vi "Data Listener.vi"(8 "error in":errorcluster, 10 "Data":T1, 11 "Connection ID":u64) -> (0 "error out":errorcluster)   [LabVIEW 2015, in "Front Panel Publisher.lvlib" / "Websocket.lvclass"]
uses:
  Websocket.lvclass
  Private/Connection Data.ctl
  Private/Mask.vi
  <vilib>/wsapi/VIs/Unescape HTTP URL.vi
  Front Panel Manager_class/FP Server Set Data.vi
  Front Panel Manager_class/FP Server Get Data.vi
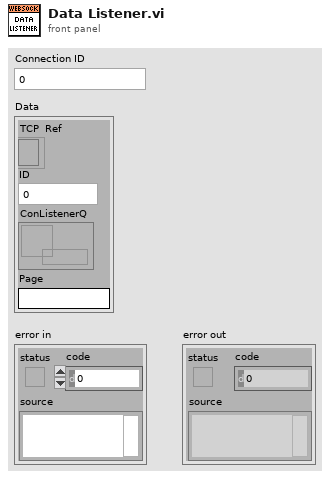
[diagram p1: front panel]
types:
  T1 = typedef "Front Panel Publisher.lvlib/Websocket.lvclass/Connection Data.ctl" = cluster{"TCP  Ref":refnum<k5>, "connection ID":u64, "ConListenerQ":refnum<queue>, "Page":string}
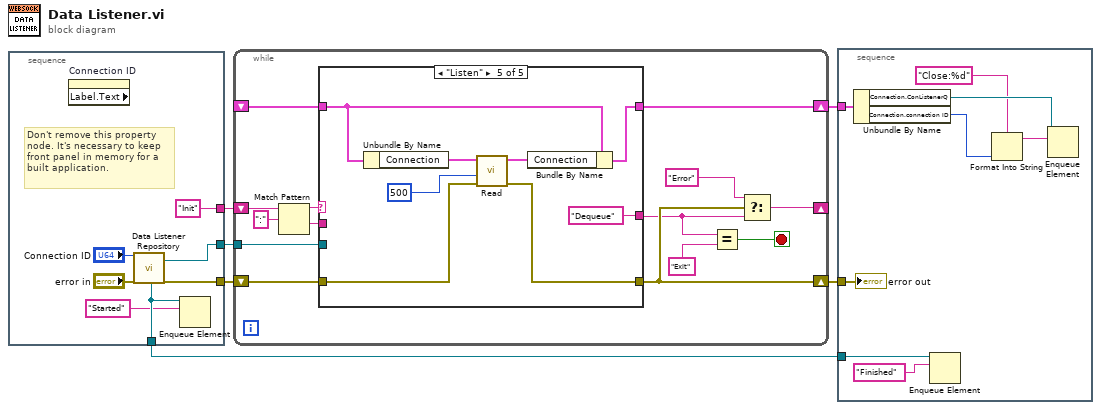
[diagram p0: block diagram]
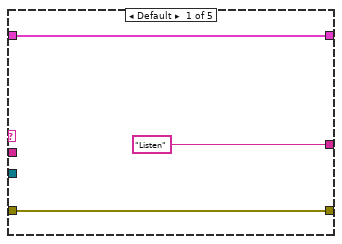
[diagram p2: hidden frame]
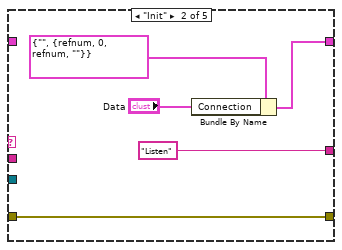
[diagram p3: hidden frame]
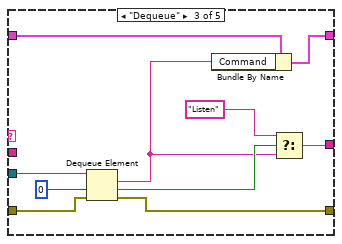
[diagram p4: hidden frame]
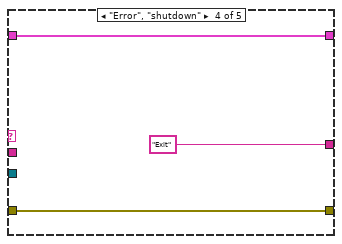
[diagram p5: hidden frame]
diagram:
  n1 = stacked-sequence {
    tunnel: [w11] -> w6
    tunnel: [w10] -> w4
    tunnel: [w8] -> w3
    tunnel: ["Init"] -> w2
    frame #0 {
      # "Don't remove this property node. It's necessary to keep front panel in memory for a built application."
      n2 = property on="Connection ID" class="DigNum (strict)" props=["Label", "Text"]() -> ()  [unwired: 2 in, 3 out]
      n3 = call "Data Listener Repository.vi"("Connection ID"="Connection ID", "error in (no error)"="error in") -> ("ProcessSyncQueue"=w8:refnum<queue>, "ToProcessQueue"=w10:refnum<queue>, "error out"=w11:errorcluster)  [unwired: 12 in, 3 out]
      n4 = Enqueue Element(queue=w8, element="Started") -> ()  [unwired: 2 in, 3 out]
    }
  }
  n5 = while {
    shift-right: [w22] -> w5
    shift-left: w6 -> [w14]
    tunnel: w4 -> [w27]
    shift-right: [w20] -> _
    shift-left: w2 -> [w25]
    shift-right: [w16] -> w1
    shift-left: _ -> [w15]
    stop <- w17 stop-if-true
    n6 = Match Pattern(string=w25, regular expression=":") -> (before substring=w24:string, after substring=w23:string)  [unwired: 1 in, 2 out]
    n7 = case shown="\"Listen\"" w24 {
      tunnel: w14 -> [w30 w33 w44 w48 w54]
      tunnel: [w30 w33 w43 w48 w53] -> w22
      tunnel: w27 -> [_ _ w45 _ _]
      tunnel: w23 -> [_ _ _ _ _]
      tunnel: ["Listen" ("t") "Listen" ("t") w40 "Exit" ("y") "Dequeue" ("t")] -> w19
      tunnel: [w28 w34 w38 w46 w50] -> w16
      tunnel: w15 -> [w28 _ w37 w46 w51]
      frame Default {
      }
      frame "Init" {
        n8 = Bundle By Name(cluster=cluster{"Command":string, "Connection":T1} {"Command"="", "Connection"={"TCP  Ref"=refnum, "connection ID"=0, "ConListenerQ"=refnum, "Page"=""}}, "Connection"="Data") -> (w34:cluster{"Command":string, "Connection":T1})
      }
      frame "Dequeue" {
        n9 = Dequeue Element(queue=w45, timeout in ms (-1)=0, error in (no error)=w44) -> (element=w39:string, timed out?=w42:bool, error out=w43:errorcluster)  [unwired: 1 out]
        n10 = Bundle By Name(cluster=w37, "Command"=w39) -> (w38:cluster{"Command":string, "Connection":T1})
        n11 = Select(t="Listen", s=w42, f=w39) -> (s? t:f=w40:string)
      }
      frame "Error", "shutdown" {
      }
      frame "Listen" {
        n12 = Unbundle By Name(w51) -> ("Connection"=w55:T1)
        n13 = call "Read.vi"("error in (no error)"=w54, "Timeout (0ms)"=500 ("timeout ms"), "Connection Data"=w55) -> ("error out"=w53:errorcluster, "Connection Data out"=w49:T1)  [unwired: 7 in]
        n14 = Bundle By Name(cluster=w51, "Connection"=w49) -> (w50:cluster{"Command":string, "Connection":T1})
      }
    }
    n15 = Equal?(x=w19, y="Exit") -> (x = y?=w17:bool)
    n16 = Select(t="Error", s=w22, f=w19) -> (s? t:f=w20:string)
  }
  n17 = stacked-sequence {
    tunnel: w5 -> [w64]
    tunnel: w3 -> [w63]
    tunnel: w1 -> [w61]
    frame #0 {
      n18 = Unbundle By Name(w61) -> ("Connection.ConListenerQ"=w60:refnum<queue>, "Connection.connection ID"=w58:u64)
      n19 = Enqueue Element(queue=w63, element="Finished") -> ()  [unwired: 2 in, 3 out]
      n20 = Format Into String(format string="Close:%d", w58) -> (resulting string=w57:string)  [unwired: 2 in, 1 out]
      n21 = Enqueue Element(queue=w60, element=w57) -> ()  [unwired: 2 in, 3 out]
      "error out" <- w64
    }
  }
